vi "LinxUartClose.vi"(8 "Error In":errorcluster, 10 "Uart Channel":u8, 11 "LINX Resource":T1) -> (0 "Error Out":errorcluster, 3 "LINX Resource":T1)   [LabVIEW 2020, in "LMH-LINX.lvlib" / "Local IO.lvlib"]
uses:
  Local IO.lvlib
  Type Defs/LINX Ref.ctl
  Type Defs/Platform.ctl
  Device/Type Defs/LINX Device Config.ctl
  Type Defs/Interface.ctl
  Device/Type Defs/TCP Config.ctl
  Device/Type Defs/Channels.ctl
  Type Defs/Error Type.ctl
  LMH-LINX.lvlib
  Type Defs/Channel FGV States.ctl
  Resources/liblinxdevice.dll
  Device/Device.lvlib
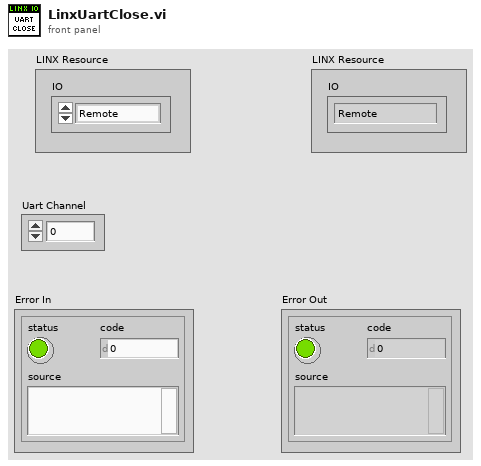
[diagram p1: front panel]
types:
  T1 = typedef "LMH-LINX.lvlib/LINX Ref.ctl" = cluster{"IO":T2, "LINX Device Config":T3}
  T2 = typedef "LMH-LINX.lvlib/Platform.ctl" = enum16{"Remote", "Local"}
  T3 = typedef "Device.lvlib/LINX Device Config.ctl" = cluster{"Interface":T4, "COM Port":refnum<visa-resource-name>, "TCP Configuration":T5, "Device Family":u8, "Device ID":u8, "Device Name":string, "TCP Ref":refnum<k5>, "Local Refnum":u64, "Channels":T6}
  T4 = typedef "LMH-LINX.lvlib/Interface.ctl" = enum16{"Serial", "TCP"}
  T5 = typedef "Device.lvlib/TCP Config.ctl" = cluster{"IP Address":string, "Port":u16}
  T6 = typedef "LMH-LINX.lvlib/Channels.ctl" = cluster{"DI":u8[], "DO":u8[], "AI":u8[], "AO":u8[], "PWM":u8[], "QE":u8[], "UART":u8[], "I2C 2":u8[], "SPI":u8[], "CAN":u8[], "Servo":u8[], "AI Ref (V)":dbl, "AI Resolution (Bits)":u8, "AO Ref (V)":dbl, "AO Resolution (Bits)":u8}
  T7 = typedef "LMH-LINX.lvlib/Error Type.ctl" = enum16{"Unknown", "Timeout", "Corrupt Return Packet", "Unable To Connect", "Command Not Supported", "Channel DNE", "Invalid COM Config", "Firmware Version Mismatch", "myRIO Support", "CMD Specific Error", "Local IO Not Supported"}
  T8 = typedef "LMH-LINX.lvlib/Channel FGV States.ctl" = enum16{"Initialize", "Get", "Set"}
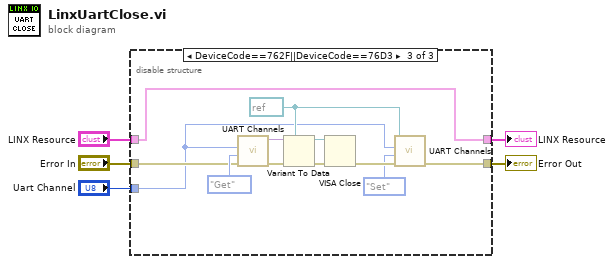
[diagram p0: block diagram]
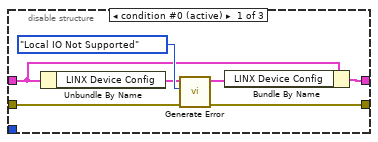
[diagram p2: hidden frame]
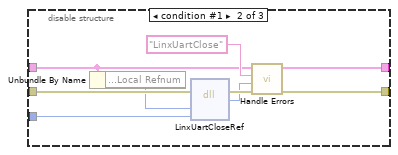
[diagram p3: hidden frame]
diagram:
  n1 = disable-structure shown="DeviceCode==762F||DeviceCode==76D3" {
    disable-tunnel: [w6 w19 w24] -> w4
    disable-tunnel: "LINX Resource" -> [w8 w13 w24]
    disable-tunnel: "Error In" -> [w11 w21 w23]
    disable-tunnel: [w10 w17 w25] -> w5
    disable-tunnel: "Uart Channel" -> [_ w20 w22]
    frame condition #0 (active) {
      n2 = Unbundle By Name(w8) -> ("LINX Device Config"=w9:T3)
      n3 = call "Generate Error.vi"("Error In"=w11, "Error Type"=Error_Type."Local IO Not Supported", "LINX Device Config"=w9) -> ("Error Out"=w10:errorcluster, "Dup LINX Device Config"=w7:T3)  [unwired: 7 in]
      n4 = Bundle By Name(cluster=w8, "LINX Device Config"=w7) -> (w6:T1)
    }
    frame condition #1 {
      n5 = Unbundle By Name(w13) -> ("LINX Device Config.Local Refnum"=w14:u64)
      n6 = dll-call lib="C:/Users/rkalbermatter/Projects/LabVIEW Hobbyist/LabVIEW/vi.lib/MakerHub/LINX/Resources/liblinxdevice.*" fn="LinxUartCloseRef"(error in=w21, "refnum"=w14, "channel"=w20) -> (error out=w18:errorcluster, "status"=w15:i32)  [unwired: 4 in, 1 out]
      n7 = call "Handle Errors.vi"("Error In"=w18, "LinxStatus"=w15, "Function Name"="LinxUartClose", "LINX Resource"=w13) -> ("Error Out"=w17:errorcluster, "LINX Resource"=w19:T1)  [unwired: 6 in]
    }
    frame condition #2 {
      w33 = refnum<visa-resource-name> refnum ("VISA resource name")
      n8 = call "UART Channels.vi"("Error In"=w23, "Channel State"=Channel_FGV_States."Get", "Channel Number"=w22) -> ("Error Out"=w29:errorcluster, "UART Channel"=w30:variant)  [unwired: 7 in]
      n9 = Variant To Data(error in=w29, type=w33, Variant=w30) -> (data=w31:refnum<visa-resource-name>, error out=w28:errorcluster)
      n10 = VISA Close(VISA resource name=w31, error in (no error)=w28) -> (error out=w32:errorcluster)
      n11 = call "UART Channels.vi"("Error In"=w32, "Channel State"=Channel_FGV_States."Set", "Channel Number"=w22, "UART Channel"=w33) -> ("Error Out"=w25:errorcluster)  [unwired: 6 in, 1 out]
    }
  }
  "LINX Resource" <- w4
  "Error Out" <- w5
